vi "Load.vi"(8 "error in (no error)":errorcluster, 10 "ID":string, 11 "Session in":refnum<class "Session.lvclass">) -> (0 "error out":errorcluster, 3 "Session out":refnum<class "Session.lvclass">)   [LabVIEW 2020, in "HTTP Server.lvlib" / "Session.lvclass"]
uses:
  Session.lvclass
  Session.lvclass/Session.ctl
  <vilib>/IlluminatedG/lv-web-crypto/lv-base64/Encode.vi
  <vilib>/IlluminatedG/lv-web-crypto/lv-crypto/Crypto/Hashes/SHA-256/SHA-256.lvclass
  <vilib>/IlluminatedG/lv-web-crypto/lv-json/JSON/JSON.lvlib
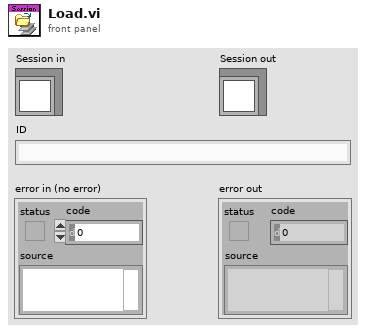
[diagram p1: front panel]
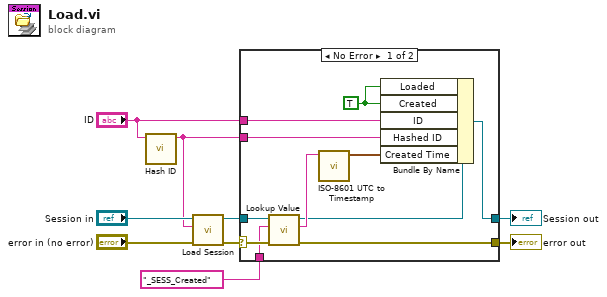
[diagram p0: block diagram]
diagram:
  n1 = call "Hash ID.vi"("ID"="ID") -> ("Hashed ID"=w4:string)  [unwired: 10 in]
  n2 = call-dynamic "Load Session.vi"("error in (no error)"="error in (no error)", "Hashed ID"=w4, "Session in"="Session in") -> ("error out"=w7:errorcluster, "Session out"=w6:refnum<class "Session.lvclass">)  [unwired: 7 in]
  n3 = case shown="No Error" w7 {
    selector: w7 -> [w15 w21]
    tunnel: w6 -> [w16 w22]
    tunnel: "ID" -> [w19 _]
    tunnel: w4 -> [w20 _]
    tunnel: [w18 w22] -> w3
    tunnel: [w10 w21] -> w2
    tunnel: "_SESS_Created" ("Name") -> [w14 _]
    frame No Error {
      w17 = TRUE ("Created")
      n4 = call "Lookup Value.vi"("error in (no error)"=w15, "Name"=w14, "Session in"=w16) -> ("error out"=w10:errorcluster, "Value"=w13:string, "Session out"=w12:refnum<class "Session.lvclass">)  [unwired: 5 in, 1 out]
      n5 = call <vilib>:"ISO-8601 UTC to Timestamp.vi"("ISO-8601"=w13) -> ("time stamp"=w11:timestamp)  [unwired: 9 in, 1 out]
      n6 = Bundle By Name(cluster=w12, "Loaded"=w17, "Created"=w17, "ID"=w19, "Hashed ID"=w20, "Created Time"=w11) -> (w18:refnum<class "Session.lvclass">)
    }
    frame Error {
    }
  }
  "error out" <- w2
  "Session out" <- w3
